vi "Write content-encoding.vi"(8 "error in (no error)":errorcluster, 10 "content-encoding":string, 11 "TCPPacket in":refnum<class "TCPPacket.lvclass">) -> (0 "error out":errorcluster, 3 "TCPPacket out":refnum<class "TCPPacket.lvclass">)   [LabVIEW 2019, in "TCPPacket.lvclass"]
uses:
  TCPPacket.lvclass
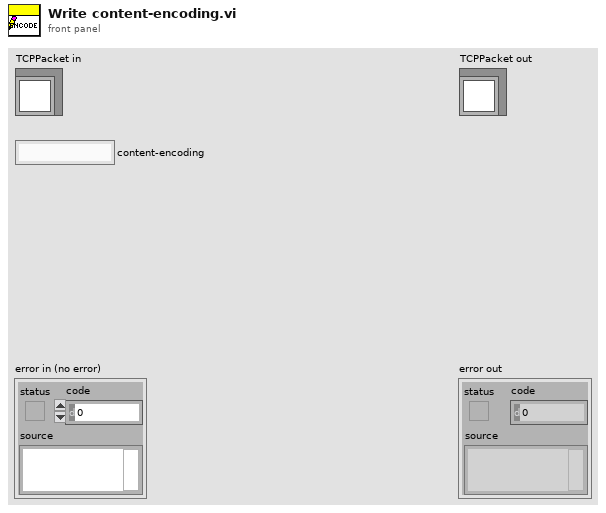
[diagram p1: front panel]
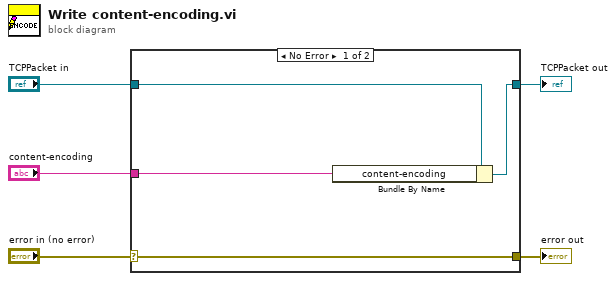
[diagram p0: block diagram]
diagram:
  n1 = case shown="No Error" "error in (no error)" {
    selector: "error in (no error)" -> [w9 w10]
    tunnel: [w9 w10] -> w4
    tunnel: [w7 w11] -> w2
    tunnel: "TCPPacket in" -> [w8 w11]
    tunnel: "content-encoding" -> [w6 _]
    frame No Error {
      n2 = Bundle By Name(cluster=w8, "content-encoding"=w6) -> (w7:refnum<class "TCPPacket.lvclass">)
    }
    frame Error {
    }
  }
  "error out" <- w4
  "TCPPacket out" <- w2
